vi "MyFPGA PWM Clock Divider.vi"(8 "Clock Select":fxp<+,3,3>) -> (2 "Enable":bool=TRUE, 3 "Reset":bool=TRUE)   [LabVIEW 2019]
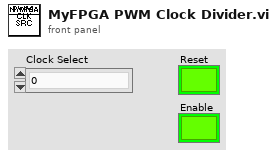
[diagram p1: front panel]
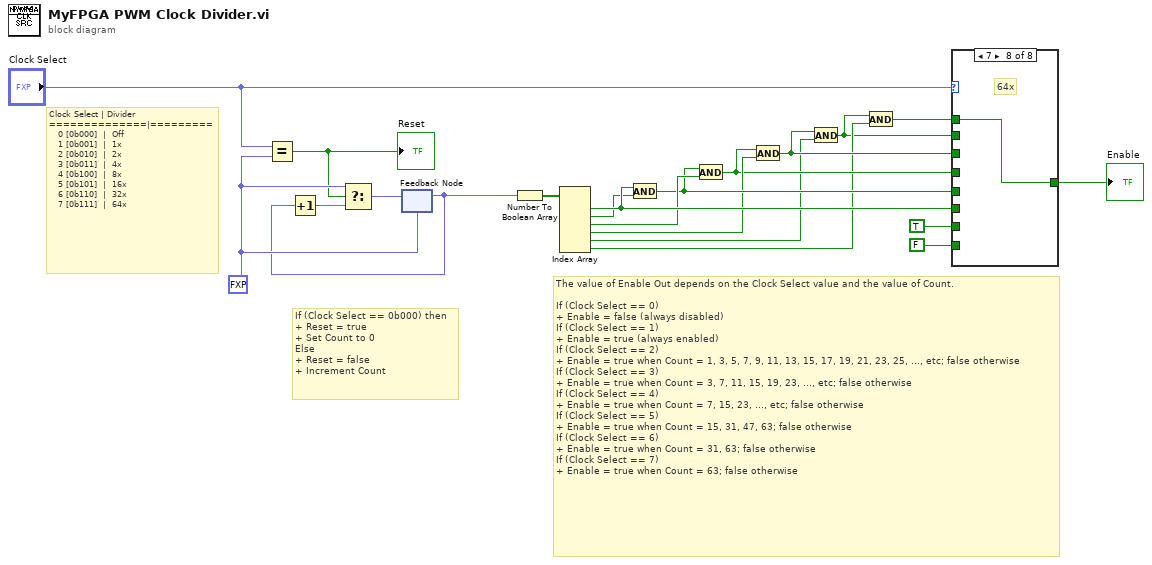
[diagram p0: block diagram]
diagram:
  w19 = fxp<+,6,6> 0.0 ("y")
  # "The value of Enable Out depends on the Clock Select value and the value of Count.\n\nIf (Clock Select == 0)\n+ Enable = false (always disabled)\nIf (Clock Select == 1)\n+ Enable = true (always enabled)\nIf (Clock Select == 2)\n+ Enable = true when Count = 1, 3, 5, 7, 9, 11, 13, 15, 17, 19, 21, 23, 25, ..., etc; false otherwise\nIf (Clock Select == 3)\n+ Enable = true when Count = 3, 7, 11, 15, 19, 23, ..., etc; false otherwise\nIf (Clock Select == 4)\n+ Enable = true when Count = 7, 15, 23, ..., etc; false otherwise\nIf (Clock Select == 5)\n+ Enable = true when Count = 15, 31, 47, 63; false otherwise\nIf (Clock Select == 6)\n+ Enable = true when Count = 31, 63; false otherwise\nIf (Clock Select == 7)\n+ Enable = true when Count = 63; false otherwise"
  # "If (Clock Select == 0b000) then\n+ Reset = true\n+ Set Count to 0\nElse\n+ Reset = false\n+ Increment Count"
  # "Clock Select | Divider \n==============|=========\n   0 [0b000]  |  Off\n   1 [0b001]  |  1x\n   2 [0b010]  |  2x\n   3 [0b011]  |  4x\n   4 [0b100]  |  8x\n   5 [0b101]  |  16x\n   6 [0b110]  |  32x\n   7 [0b111]  |  64x"
  n1 = Equal?(x="Clock Select", y=w19) -> (x = y?=w17:bool)
  "Reset" <- w17
  n2 = feedback #1(w19) -> (w16:fxp<+,6,6>)
  n3 = Increment(x=w16) -> (x+1=w18:fxp<+,6,6>)
  n4 = Select(t=w19, s=w17, f=w18) -> (s? t:f=w20:fxp<+,6,6>)
  n5 = feedback-in #1(w20) -> ()
  n6 = Number To Boolean Array(number=w16) -> (Boolean array=w14:bool[])
  n7 = Index Array(array=w14) -> (element #1=w13:bool, element #2=w12:bool, element #3=w11:bool, element #4=w7:bool, element #5=w4:bool, element #6=w3:bool)  [unwired: 6 in]
  n8 = And(x=w13, y=w12) -> (x .and. y?=w10:bool)
  n9 = And(x=w10, y=w11) -> (x .and. y?=w6:bool)
  n10 = And(x=w6, y=w7) -> (x .and. y?=w5:bool)
  n11 = And(x=w5, y=w4) -> (x .and. y?=w2:bool)
  n12 = And(x=w2, y=w3) -> (x .and. y?=w1:bool)
  n13 = case shown="7" "Clock Select" {
    tunnel: [w22 w23 w24 w25 w26 w27 w28 w29] -> w15
    tunnel: w13 -> [_ _ w24 _ _ _ _ _]
    tunnel: w10 -> [_ _ _ w25 _ _ _ _]
    tunnel: w6 -> [_ _ _ _ w26 _ _ _]
    tunnel: TRUE -> [_ w23 _ _ _ _ _ _]
    tunnel: FALSE -> [w22 _ _ _ _ _ _ _]
    tunnel: w5 -> [_ _ _ _ _ w27 _ _]
    tunnel: w2 -> [_ _ _ _ _ _ w28 _]
    tunnel: w1 -> [_ _ _ _ _ _ _ w29]
    frame 0, Default {
      # "None"
    }
    frame 1 {
      # "1x"
    }
    frame 2 {
      # "2x"
    }
    frame 3 {
      # "4x"
    }
    frame 4 {
      # "8x"
    }
    frame 5 {
      # "16x"
    }
    frame 6 {
      # "32x"
    }
    frame 7 {
      # "64x"
    }
  }
  "Enable" <- w15
